vi "niDTS Comm String Send Script.vi"(0 "Comm String Handle":T1, 5 "Script":string, 11 "error in (no error)":errorcluster) -> (4 "Comm String Handle Out":T1, 6 "Return":string, 15 "error out":errorcluster)   [LabVIEW 2015, in "niDTS CommLib.lvlib"]
doc: "This sends the Command concatenated with the Args over the String Interface.\n\nInputs:\n* Command (Required): This is the command to be sent.\n* Args (Optional): Any arguments to be concatenated with the command.\n\nOutputs:\n* Response: Any data returned from the interface. Note that no data wil be returned if the flag Read Enabled is set to FALSE."
uses:
  niDTS CommLib.lvlib
  Includes/niDTS Comm String INC Handle.ctl
  Objects/String_class/niDTS Comm String.lvclass
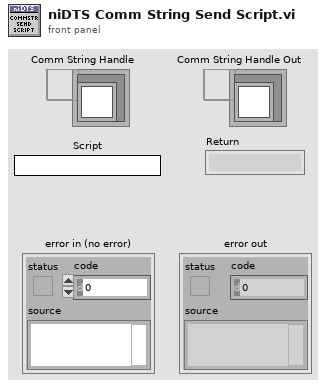
[diagram p1: front panel]
types:
  T1 = typedef "niDTS CommLib.lvlib/niDTS Comm String INC Handle.ctl" = refnum<data-value>
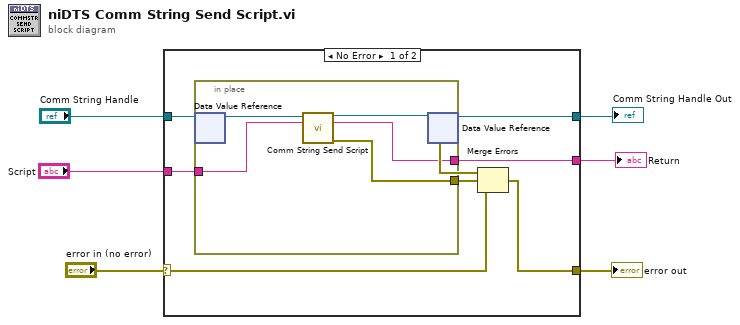
[diagram p0: block diagram]
diagram:
  n1 = case shown="No Error" "error in (no error)" {
    selector: "error in (no error)" -> [w12 w21]
    tunnel: [w11 w21] -> w6
    tunnel: "Comm String Handle" -> [w14 w20]
    tunnel: [w10 w20] -> w3
    tunnel: "Script" -> [w8 _]
    tunnel: [w7 _] -> w1
    frame No Error {
      n2 = in-place {
        in-place-border: [w18] -> w9
        in-place-border: w8 -> [w17]
        in-place-border: [w15] -> w7
        n3 = in-place-dvr #1(w14) -> (w19:refnum<class "niDTS Comm String.lvclass">)  [unwired: 1 out]
        n4 = call-dynamic "Comm String Send Script.vi"("niDTS Comm String in"=w19, "script"=w17) -> ("niDTS Comm String out"=w16:refnum<class "niDTS Comm String.lvclass">, "Return"=w15:string, "error out"=w18:errorcluster)  [unwired: 11 in]
        n5 = in-place-dvr #1(w16) -> (w10:T1, w13:errorcluster)
      }
      n6 = Merge Errors(w13, w9, w12) -> (w11:errorcluster)
    }
    frame Error {
    }
  }
  "error out" <- w6
  "Comm String Handle Out" <- w3
  "Return" <- w1
